vi "Close.vi"(8 "error in (no error)":errorcluster, 11 "Power Supply Instrument in":refnum<class "Power Supply Instrument.lvclass">) -> (0 "error out":errorcluster, 3 "Power Supply Instrument out":refnum<class "Power Supply Instrument.lvclass">)   [LabVIEW 2025, in "Power Supply.lvlib" / "Power Supply Instrument.lvclass"]
uses:
  Power Supply Instrument.lvclass
  Power Supply Instrument.lvclass/Power Supply Instrument.ctl
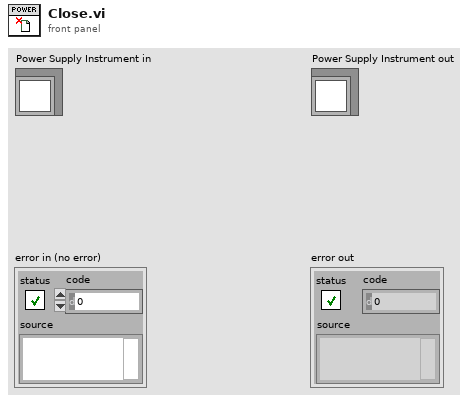
[diagram p1: front panel]
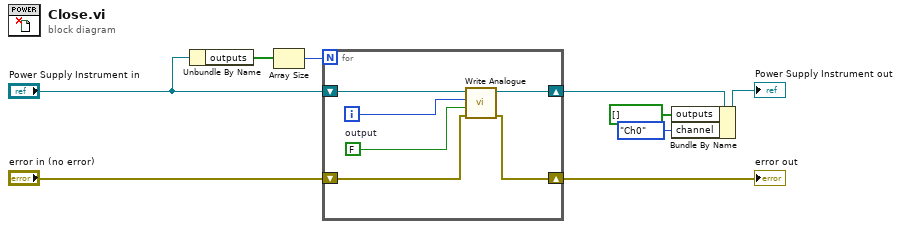
[diagram p0: block diagram]
diagram:
  n1 = Unbundle By Name("Power Supply Instrument in") -> ("outputs"=w2:bool[])
  n2 = Array Size(array=w2) -> (size(s)=w1:i32)
  n3 = for {
    N: w1 -> [_]
    shift-right: [w14] -> w5
    shift-left: "error in (no error)" -> [w15]
    shift-right: [w12] -> w4
    shift-left: "Power Supply Instrument in" -> [w13]
    i -> [w10]
    w11 = FALSE  # output
    n4 = call-dynamic "Write Analogue.vi"("error in (no error)"=w15, "output"=w11, "Channel index"=w10, "PS Instrument"=w13) -> ("error out"=w14:errorcluster, "PS Instrument out"=w12:refnum<class "Power Supply Instrument.lvclass">)  [unwired: 5 in, 1 out]
  }
  "error out" <- w5
  n5 = Bundle By Name(cluster=w4, "outputs"=bool[] [], "channel"=enum32{"Ch0", "Ch1", "Ch2", "Ch3"}."Ch0") -> (→"Power Supply Instrument out":refnum<class "Power Supply Instrument.lvclass">)
